vi "HDI-BBM Start Position Acquire.vi"() -> ()   [LabVIEW 2011]
uses:
  Shared Components/Orient3d Class/Type Definitions/Quaternion.ctl
  Shared Components/Config Manager Class/Type Definitions/Part Type.ctl
  Shared Components/Gantry Class/Gantry Class.lvclass
  Shared Components/Vec3d Class/Vec3d Class.lvclass
  Shared Components/Config Manager Class/Type Definitions/Camera Enum.ctl
  Shared Components/Orient3d Class/Orient3d Class.lvclass
  Shared Components/Config Manager Class/Config Manager Class.lvclass
panel:
  in  "Tab Control":enum32{"Control", "Results"}(tab)
  out "error out":errorcluster
  out "preview":T1(plugin-control)
  out "Current Position":cluster{"X":dbl, "Y":dbl, "Z":dbl}
  in  "Slot":i32=1
  in  "Capture":bool
  in  "Config Folder":path=path "C:/Users/Husker/Desktop/gantry/Config"
  in  "Chuck":i32=1
  in  "Part Type":T2
  out "Current Fiducial":string
  out "Orientation":T3
  out "Center":cluster{"X":dbl, "Y":dbl, "Z":dbl}
  out "Residual":dbl
  out "Measured Positions":cluster{"X":dbl, "Y":dbl, "Z":dbl}[](array[cluster])
  out "Known Positions":cluster{"X":dbl, "Y":dbl, "Z":dbl}[](array[cluster])
  out "Config String":string
  out "DoCapture":bool
  # "INSTRUCTIONS\n==========\nThis is a tool to help in the acquisition\nof starting(default) part positions.\n\nBegin by setting appropriate values in the \nlower left corner.\n\nThen use the MPG(hand control) to move\nto the center of the part's fiducial as indicated in the \nCurrent Fiducial field.\n\nAfter moving over a fiducial, click the \"Capture\"\nButton. \n\nAfter location all fiducials, examine the \"Results\"\nTab. Note the"
  # "Set this to the appropriate slot number(0-3) before running"
  # "Set this to the appropriate chuck number(0-4) before running"
  # "Set this to the appropriate part type (HDI, BBM, etc.) before running"
  # "Press this button after \ncentering the fiducial in the image"
  # "After aquiring positions, place these results in\npart_location.ini under the correct part heading"
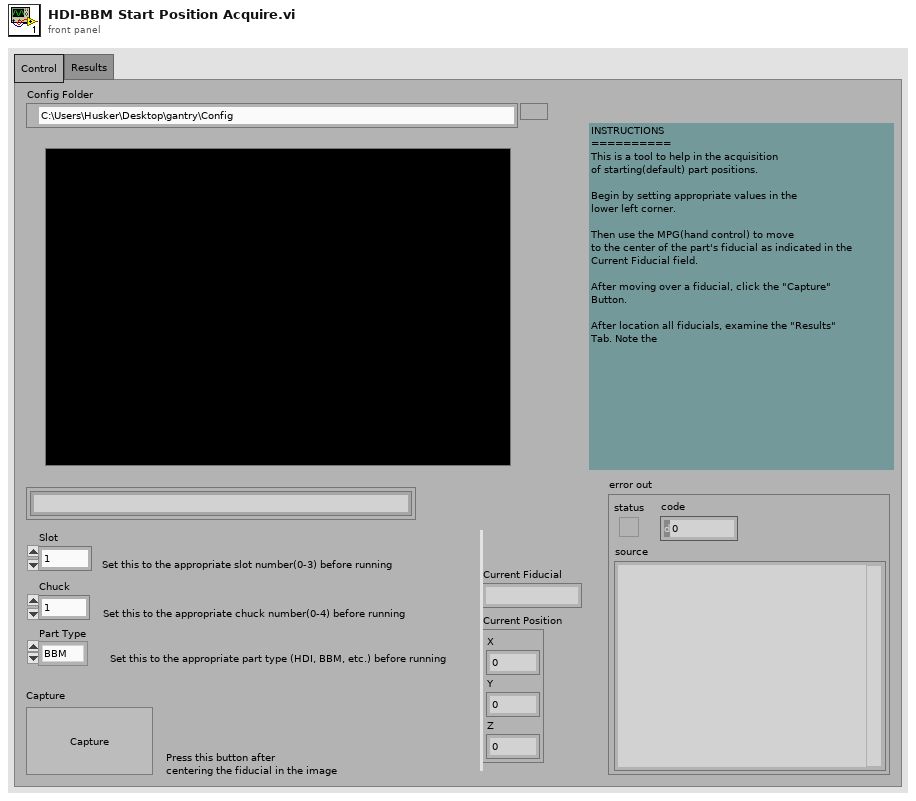
[diagram p1: front panel]
types:
  T1 = typedef "IMAQ Image.ctl" = refnum<image>
  T2 = typedef "Part Type.ctl" = enum16{"BBM", "HDI", "BARE HDI", "GLUERESERVOIR", "STAMP_1", "STAMP_2", "STAMP_3", "STAMP_4", "STAMP_5", "WEIGHT_1", "WEIGHT_2", "WEIGHT_3", "WEIGHT_4", "WEIGHT_5", "WEIGHT_6", "WEIGHT_7", "WEIGHT_8", "PICKER_TOOL", "GRABER_TOOL"}
  T3 = typedef "Quaternion.ctl" = cluster{"x":dbl, "y":dbl, "z":dbl, "w":dbl}
  T4 = typedef "Fiducial Type.ctl" = enum16{"HDI", "BBM"}
  T5 = cluster{"Feature Coordinates":refnum<class "Vec3d Class.lvclass">, "Feature Name":string}[]
  T6 = typedef "Camera Enum.ctl" = enum16{"GANTRY HEAD", "NEEDLE CALIBRATION X", "NEEDLE CALIBRATION Y"}
  T7 = typedef "Image Type" = u32
  T8 = typedef "Physical Image.ctl" = cluster{"Image Position":refnum<class "Vec3d Class.lvclass">, "Image Reference":T1, "Field of View":cluster{"x(mm)":dbl, "y(mm)":dbl}}
  T9 = typedef "Position_Orientation.ctl" = cluster{"Center":refnum<class "Vec3d Class.lvclass">, "Orientation":refnum<class "Orient3d Class.lvclass">}
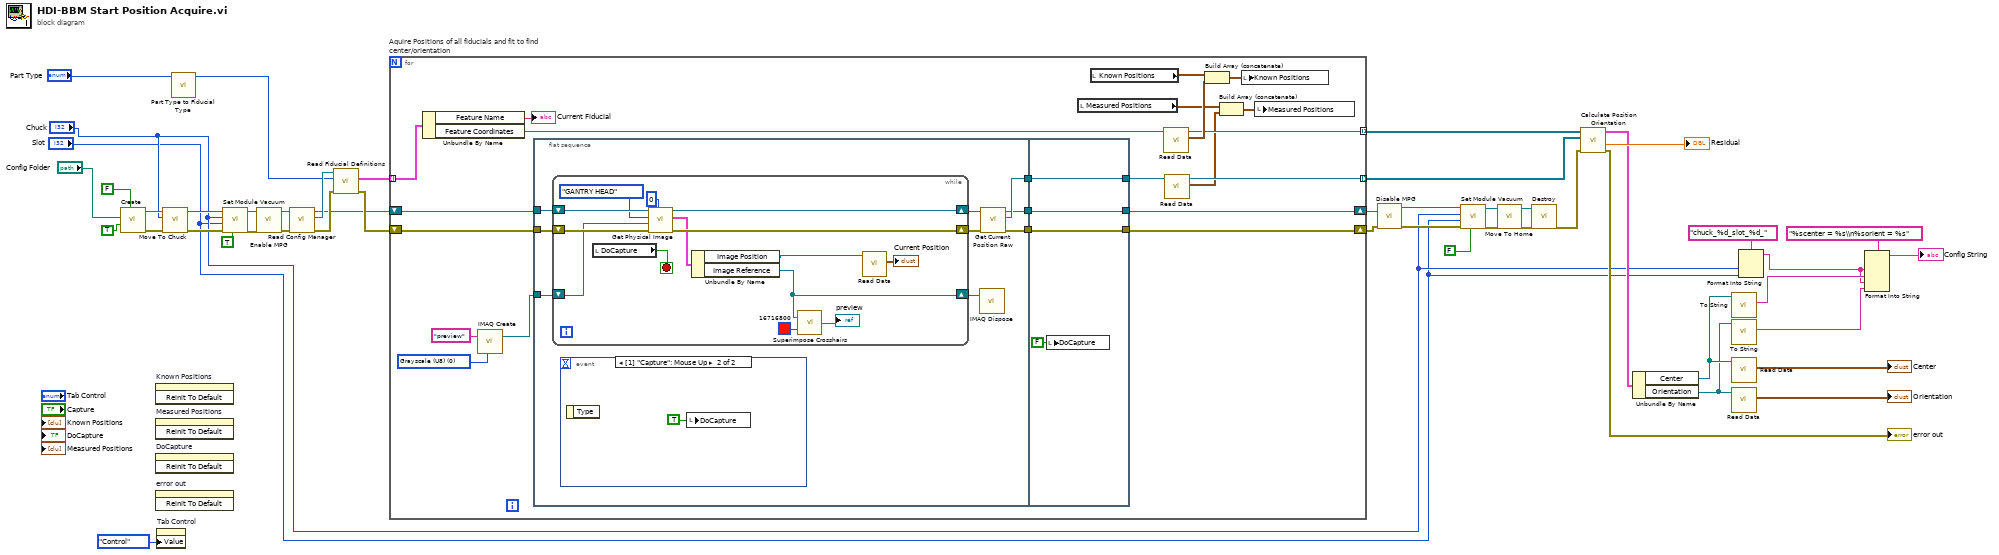
[diagram p0: block diagram]
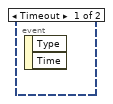
[diagram p2: hidden frame]
diagram:
  n1 = call "Create.vi"("Virtual Mode"=FALSE, "HOME?"=TRUE, "Config Folder"="Config Folder") -> ("error out"=w35:errorcluster, "Gantry out"=w33:refnum<class "Gantry Class.lvclass">)  [unwired: 7 in]
  n2 = invoke on="Known Positions" class="Arr (strict)" method="Reinit To Default"() -> ()  [unwired: 3 in, 3 out]
  n3 = invoke on="Measured Positions" class="Arr (strict)" method="Reinit To Default"() -> ()  [unwired: 3 in, 3 out]
  n4 = invoke on="DoCapture" class="Bool (strict)" method="Reinit To Default"() -> ()  [unwired: 3 in, 3 out]
  n5 = invoke on="error out" class="Clust (strict)" method="Reinit To Default"() -> ()  [unwired: 3 in, 3 out]
  n6 = property on="Tab Control" class="TabCtl (strict)"("Value"=enum32{"Control", "Results"}."Control" ("Tab Control")) -> ()  [unwired: 2 in, 2 out]
  n7 = call-dynamic "Move To Chuck.vi"("error in"=w35, "Chuck"="Chuck", "Gantry in"=w33) -> ("error out"=w34:errorcluster, "Gantry out"=w32:refnum<class "Gantry Class.lvclass">)  [unwired: 7 in]
  n8 = call "Part Type to Fiducial Type.vi"("Part Type"="Part Type") -> ("Fiducial Type"=w13:T4)  [unwired: 9 in, 1 out]
  n9 = call-dynamic "Set Module Vacuum.vi"("On/Off"=TRUE, "error in"=w34, "Slot Number"="Slot", "Chuck Number"="Chuck", "Gantry in"=w32) -> ("error out"=w43:errorcluster, "Gantry out"=w44:refnum<class "Gantry Class.lvclass">)  [unwired: 5 in]
  n10 = call-dynamic "Enable MPG.vi"("error in"=w43, "Gantry in"=w44) -> ("error out"=w16:errorcluster, "Gantry out"=w17:refnum<class "Gantry Class.lvclass">)  [unwired: 8 in]
  n11 = call-dynamic "Read Config Manager.vi"("error in"=w16, "Gantry in"=w17) -> ("error out"=w18:errorcluster, "Config Manager"=w19:refnum<class "Config Manager Class.lvclass">, "Gantry out"=w14:refnum<class "Gantry Class.lvclass">)  [unwired: 7 in]
  n12 = call "Read Fiducial Definitions.vi"("error in"=w18, "Fiducial Type"=w13, "Config Manager in"=w19) -> ("error out"=w15:errorcluster, "Feature Definitions"=w12:T5)  [unwired: 6 in, 1 out]
  n13 = for "Aquire Positions of all fiducials and fit to find center/orientation" {
    tunnel: [w61] -> w40 mode=indexing
    tunnel: [w59] -> w39 mode=indexing
    shift-right: [w69] -> w42
    shift-left: w14 -> [w55]
    shift-right: [w68] -> w41
    shift-left: w15 -> [w54]
    tunnel: w12 -> [w53] mode=indexing
    w50 = T7 0 items=["Grayscale (U8)", "Grayscale (I16)", "Grayscale (SGL)", "Complex (CSG)", "RGB (U32)", "HSL (U32)", "RGB (U64)", "Grayscale (U16)"] ("Image Type")
    n14 = Unbundle By Name(w53) -> ("Feature Name"=→"Current Fiducial":string, "Feature Coordinates"=w51:refnum<class "Vec3d Class.lvclass">)
    n15 = call "IMAQ Create"("Image Name"="preview", "Image Type"=w50) -> ("New Image"=w48:T1)  [unwired: 3 in, 1 out]
    n16 = flat-sequence {
      tunnel: w54 -> [w70]
      tunnel: [w76] -> w67
      tunnel: [w75] -> w66
      tunnel: [w74] -> w65
      tunnel: w48 -> [w73]
      tunnel: w55 -> [w71]
      tunnel: [w95] -> w68
      tunnel: [w96] -> w69
      tunnel: [w97] -> w60
      tunnel: w67 -> [w97]
      tunnel: w66 -> [w96]
      tunnel: w65 -> [w95]
      frame #0 {
        n17 = while {
          shift-right: [w85] -> w78
          shift-left: w70 -> [w91]
          shift-right: [w86] -> w77
          shift-left: w71 -> [w92]
          shift-right: [w82] -> w72
          shift-left: w73 -> [w87]
          stop <- w93 stop-if-true
          n18 = local read "DoCapture"() -> (w93:bool)
          n19 = call-dynamic "Get Physical Image.vi"("Delay(milliseconds)"=0, "error in"=w91, "Image In"=w87, "Camera Name"=Camera_Enum."GANTRY HEAD", "Gantry in"=w92) -> ("error out"=w85:errorcluster, "Physical Image"=w84:T8, "Gantry out"=w86:refnum<class "Gantry Class.lvclass">)  [unwired: 4 in]
          n20 = Unbundle By Name(w84) -> ("Image Position"=w83:refnum<class "Vec3d Class.lvclass">, "Image Reference"=w82:T1)
          n21 = call "Superimpose Crosshairs.vi"("Grid Line Color"=u32 16716800, "Refnum in"=w82) -> ("Refnum out"=→"preview":T1)
          n22 = call-dynamic "Read Data.vi"("Vec3d Class in"=w83) -> ("Data"=→"Current Position":cluster{"X":dbl, "Y":dbl, "Z":dbl})  [unwired: 8 in, 2 out]
        }
        n23 = event shown="[1] \"Capture\": Mouse Up" {
          selector: _ -> [_ _]
          dyn-events: _ -> [_ _]
          timeout: _ -> [_ _]
          event Timeout {
            n24 = event-data() -> ()  [unwired: 1 in, 2 out]
          }
          event "Capture": Mouse Up {
            n25 = event-data() -> ()  [unwired: 1 in, 1 out]
            n26 = local write "DoCapture"(TRUE ("DoCapture")) -> ()
          }
        }
        n27 = call "IMAQ Dispose"("Image"=w72) -> ()  [unwired: 5 in, 1 out]
        n28 = call-dynamic "Get Current Position Raw.vi"("error in"=w78, "Gantry in"=w77) -> ("error out"=w74:errorcluster, "Vec3d Class out"=w76:refnum<class "Vec3d Class.lvclass">, "Gantry out"=w75:refnum<class "Gantry Class.lvclass">)  [unwired: 7 in]
      }
      frame #1 {
        n29 = local write "DoCapture"(FALSE ("DoCapture")) -> ()
      }
    }
    n30 = local read "Measured Positions"() -> (w58:cluster{"X":dbl, "Y":dbl, "Z":dbl}[])
    n31 = local read "Known Positions"() -> (w64:cluster{"X":dbl, "Y":dbl, "Z":dbl}[])
    n32 = call-dynamic "Read Data.vi"("Vec3d Class in"=w51) -> ("Data"=w63:cluster{"X":dbl, "Y":dbl, "Z":dbl}, "Vec3d Class out"=w61:refnum<class "Vec3d Class.lvclass">)  [unwired: 8 in, 1 out]
    n33 = call-dynamic "Read Data.vi"("Vec3d Class in"=w60) -> ("Data"=w56:cluster{"X":dbl, "Y":dbl, "Z":dbl}, "Vec3d Class out"=w59:refnum<class "Vec3d Class.lvclass">)  [unwired: 8 in, 1 out]
    n34 = Build Array (concatenate)(w64, w63) -> (w62:cluster{"X":dbl, "Y":dbl, "Z":dbl}[])
    n35 = Build Array (concatenate)(w58, w56) -> (w57:cluster{"X":dbl, "Y":dbl, "Z":dbl}[])
    n36 = local write "Known Positions"(w62) -> ()
    n37 = local write "Measured Positions"(w57) -> ()
  }
  n38 = call-dynamic "Disable MPG.vi"("error in"=w41, "Gantry in"=w42) -> ("error out"=w29:errorcluster, "Gantry out"=w30:refnum<class "Gantry Class.lvclass">)  [unwired: 8 in]
  n39 = call-dynamic "Set Module Vacuum.vi"("On/Off"=FALSE, "error in"=w29, "Slot Number"="Slot", "Chuck Number"="Chuck", "Gantry in"=w30) -> ("error out"=w25:errorcluster, "Gantry out"=w27:refnum<class "Gantry Class.lvclass">)  [unwired: 5 in]
  n40 = call-dynamic "Move To Home.vi"("error in"=w25, "Gantry in"=w27) -> ("error out"=w24:errorcluster, "Gantry out"=w26:refnum<class "Gantry Class.lvclass">)  [unwired: 8 in]
  n41 = call "Destroy.vi"("error in"=w24, "Gantry Class in"=w26) -> ("error out"=w28:errorcluster)  [unwired: 9 in]
  n42 = call "Calculate Position Orientation.vi"("error in"=w28, "Measured Global Positions"=w39, "Known Local Positions"=w40) -> ("error out"=→"error out":errorcluster, "Residual"=→"Residual":dbl, "PositionOrientation"=w36:T9)  [unwired: 6 in]
  n43 = Unbundle By Name(w36) -> ("Center"=w11:refnum<class "Vec3d Class.lvclass">, "Orientation"=w10:refnum<class "Orient3d Class.lvclass">)
  n44 = call "To String.vi"("Vec3d in"=w11) -> ("Vec3d String"=w5:string)  [unwired: 8 in, 2 out]
  n45 = call "To String.vi"("Orient3d in"=w10) -> ("Orient3d String"=w3:string)  [unwired: 8 in, 2 out]
  n46 = call-dynamic "Read Data.vi"("Vec3d Class in"=w11) -> ("Data"=→"Center":cluster{"X":dbl, "Y":dbl, "Z":dbl})  [unwired: 8 in, 2 out]
  n47 = call "Read Data.vi"("Orient3d in"=w10) -> ("Quaternion"=→"Orientation":T3)  [unwired: 8 in, 2 out]
  n48 = Format Into String(format string="chuck_%d_slot_%d_", "Chuck", "Slot") -> (resulting string=w4:string)  [unwired: 2 in, 1 out]
  n49 = Format Into String(format string="%scenter = %s\\n%sorient = %s", w4, w5, w4, w3) -> (resulting string=→"Config String":string)  [unwired: 2 in, 1 out]
